vi "Establish Connection.vi"(6 "GenNet Protocol":refnum<class "GenNet Protocol.lvclass">, 8 "error in":errorcluster, 9 "Caller's Queue In":refnum<class "DQMH-GenNet Message Queue.lvclass">, 10 "Module ID":i32, 11 "Data Cluster":T1) -> (0 "error out":errorcluster, 3 "Data Cluster out":T1)   [LabVIEW 2020, in "GenNet-Client.lvlib"]
doc: "Opens the TCP/IP connection to the GenNet Server module and evaluates the result. \n\nThe connection parameters are stored in this module's data cluster for potential (re)connection attempts.\n\n____\nHAMPEL SOFTWARE ENGINEERING v3.8.0 (2023-12-18 14:41)"
uses:
  GenNet-Client.lvlib
  Module Data--cluster.ctl
  GenNet Protocols/GenNet Protocol.lvclass
  DQMH-GenNet Message Queue.lvclass
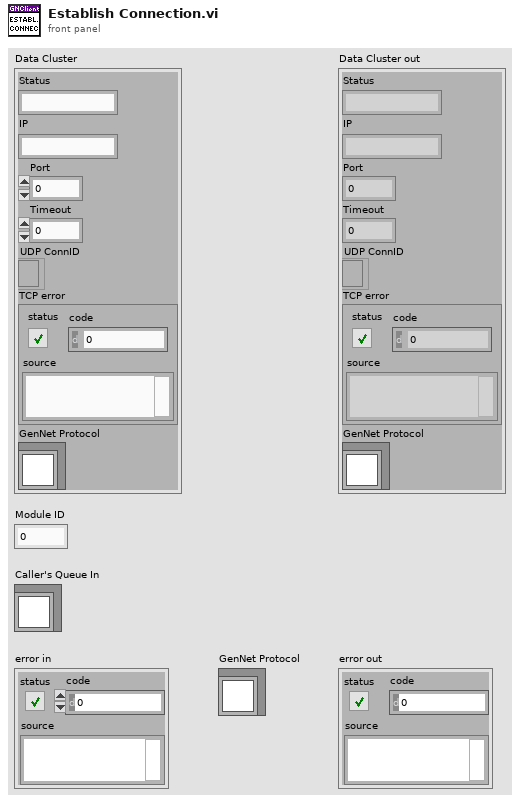
[diagram p1: front panel]
types:
  T1 = typedef "GenNet-Client.lvlib/Module Data--cluster.ctl" = cluster{"Status":string, "IP":string, "Port":u16, "Timeout":i32, "UDP ConnID":refnum<k16>, "TCP error":errorcluster, "GenNet Protocol":refnum<class "GenNet Protocol.lvclass">}
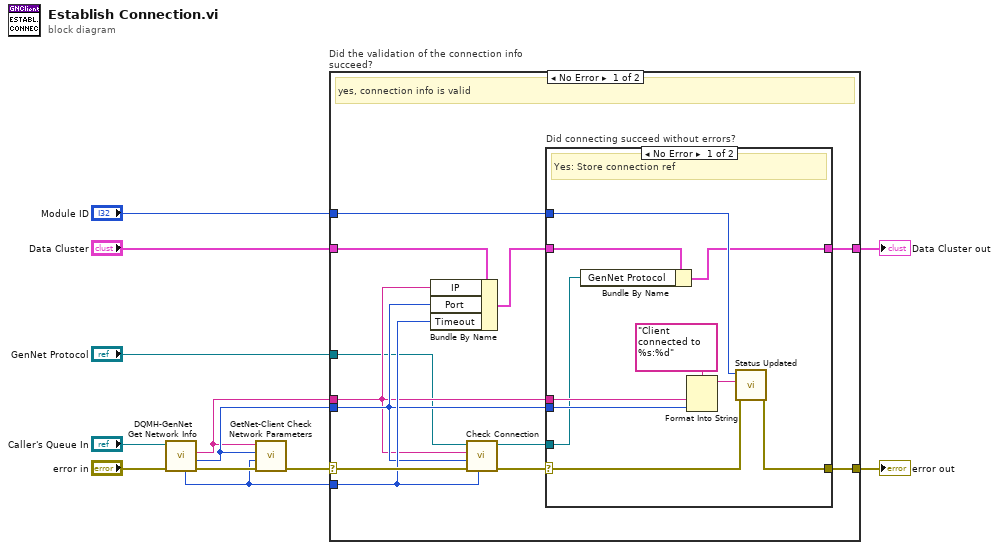
[diagram p0: block diagram]
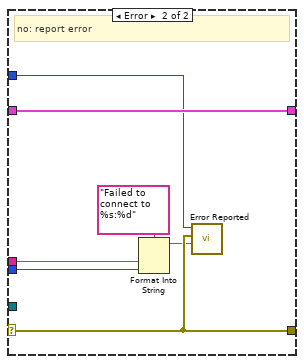
[diagram p2: hidden frame]
diagram:
  n1 = call "DQMH-GenNet Get Network Info.vi"("error in (no error)"="error in", "Message Queue in"="Caller's Queue In") -> ("error out"=w10:errorcluster, "Port Number"=w7:u16, "IP Address"=w6:string, "Timeout"=w8:i32)  [unwired: 5 in, 1 out]
  n2 = call "GetNet-Client Check Network Parameters.vi"("error in (no error)"=w10, "Timeout"=w8, "Port"=w7, "IP"=w6) -> ("error out"=w11:errorcluster)  [unwired: 7 in]
  n3 = case "Did the validation of the connection info succeed?" shown="No Error" w11 {
    selector: w11 -> [w23 w42]
    tunnel: "Data Cluster" -> [w24 w43]
    tunnel: w8 -> [w22 _]
    tunnel: w7 -> [w20 _]
    tunnel: w6 -> [w19 _]
    tunnel: "Module ID" -> [w17 _]
    tunnel: [w15 w43] -> w4
    tunnel: [w14 w42] -> w3
    tunnel: "GenNet Protocol" -> [w13 _]
    frame No Error {
      # "yes, connection info is valid"
      n4 = Bundle By Name(cluster=w24, "IP"=w19, "Port"=w20, "Timeout"=w22) -> (w18:T1)
      n5 = call-dynamic "Check Connection.vi"("timeout [ms]"=w22, "error in (no error)"=w23, "remote port"=w20, "ip address"=w19, "GenNet Protocol in"=w13) -> ("error out"=w21:errorcluster, "GenNet Protocol out"=w16:refnum<class "GenNet Protocol.lvclass">)  [unwired: 5 in]
      n6 = case "Did connecting succeed without errors?" shown="No Error" w21 {
        selector: w21 -> [w27 w36]
        tunnel: w17 -> [w33 w40]
        tunnel: w16 -> [w28 _]
        tunnel: w19 -> [w32 w38]
        tunnel: w20 -> [w31 w37]
        tunnel: [w25 w36] -> w14
        tunnel: [w29 w41] -> w15
        tunnel: w18 -> [w30 w41]
        frame No Error {
          # "Yes: Store connection ref"
          n7 = Bundle By Name(cluster=w30, "GenNet Protocol"=w28) -> (w29:T1)
          n8 = Format Into String(format string="Client connected to %s:%d", w32, w31) -> (resulting string=w26:string)  [unwired: 2 in, 1 out]
          n9 = call "Status Updated.vi"("error in (no error)"=w27, "Status"=w26, "Module ID"=w33) -> ("error out"=w25:errorcluster)  [unwired: 8 in]
        }
        frame Error {
          # "no: report error"
          n10 = Format Into String(format string="Failed to connect to %s:%d", w38, w37) -> (resulting string=w35:string)  [unwired: 2 in, 1 out]
          n11 = call "Error Reported.vi"("Additional Information"=w35, "Error"=w36, "Module ID"=w40) -> ()  [unwired: 8 in, 1 out]
        }
      }
    }
    frame Error {
      # "No, connection info is not valid"
    }
  }
  "Data Cluster out" <- w4
  "error out" <- w3
